vi "Error Query.vi"(8 "error in (no error)":errorcluster, 11 "VISA resource name":refnum<visa-resource-name>) -> (0 "error out":errorcluster, 1 "Error Message":string, 2 "Error Code":i32[](array[numeric]), 3 "VISA resource name out":refnum<visa-resource-name>)   [LabVIEW 2013]
doc: "This VI queries the instrument for any errors in the instrument's error queue. It will continue to read errors until all errors have been read from the instrument. Any errors will be returned in the Error Out cluster.\n\nNote:\nThis VI is called automatically by most driver VIs so it is not usually necessary to call this in an application."
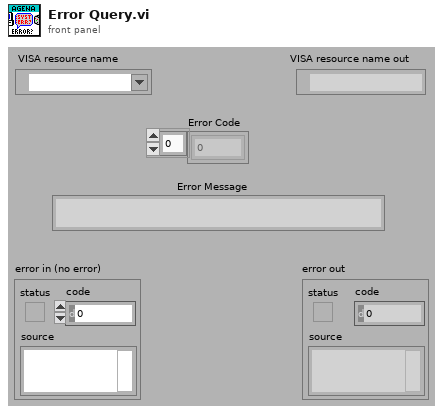
[diagram p1: front panel]
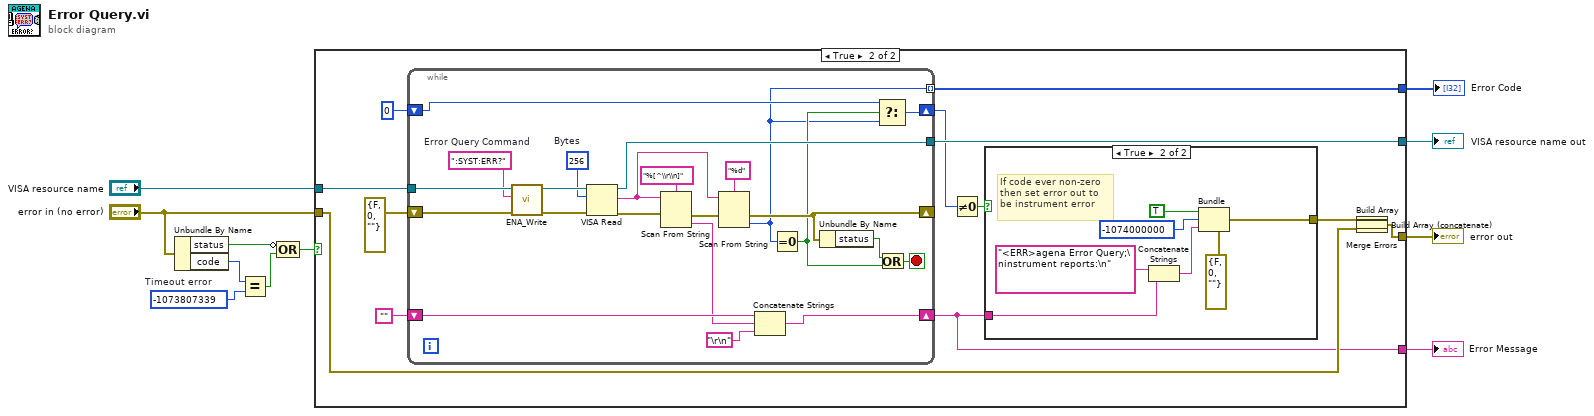
[diagram p0: block diagram]
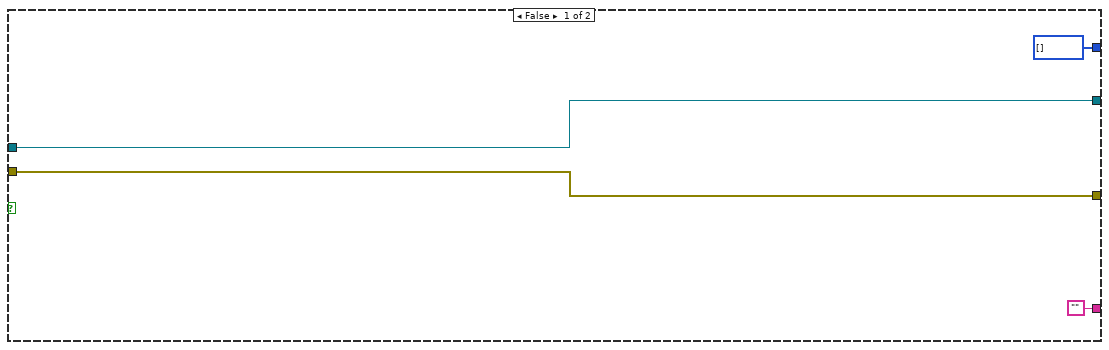
[diagram p2: hidden frame]
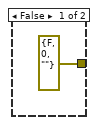
[diagram p3: hidden frame]
diagram:
  w6 = -1073807339  # Timeout error
  n1 = Unbundle By Name("error in (no error)") -> ("status"=w7:bool, "code"=w4:i32)
  n2 = Equal?(x=w4, y=w6) -> (x = y?=w5:bool)
  n3 = Compound Arithmetic op=OR(invert w7, w5) -> (w3:bool)
  n4 = case shown="True" w3 {
    tunnel: [w15 w29] -> w11
    tunnel: "VISA resource name" -> [w15 w28]
    tunnel: "error in (no error)" -> [w14 w22]
    tunnel: [w14 w26] -> w9
    tunnel: ["" w19] -> w2
    tunnel: [i32[] [] w18] -> w1
    frame False {
    }
    frame True {
      n5 = while {
        tunnel: [w60] -> w29
        tunnel: w28 -> [w59]
        shift-right: [w47] -> w19
        shift-left: "" -> [w50]
        shift-right: [w45] -> w20
        shift-left: 0 -> [w46]
        shift-right: [w43] -> _
        shift-left: errorcluster {"status"=FALSE, "code"=0, "source"=""} ("error in (no error)") -> [w44]
        tunnel: [w38] -> w18 mode=indexing
        stop <- w53 stop-if-true
        w57 = u32 256  # Bytes
        w55 = ":SYST:ERR?"  # Error Query Command
        n6 = call "ENA_Write.vi"("error in (no error)"=w44, "String ()"=w55, "VISA resource name"=w59) -> ("error out"=w56:errorcluster, "VISA resource name out"=w58:refnum<visa-resource-name>)  [unwired: 6 in, 1 out]
        n7 = VISA Read(VISA resource name=w58, byte count=w57, error in (no error)=w56) -> (VISA resource name out=w60:refnum<visa-resource-name>, read buffer=w51:string, error out=w42:errorcluster)  [unwired: 1 out]
        n8 = Scan From String(format string="%[^\\r\\n]", input string=w51, error in=w42) -> (error out=w41:errorcluster, output 1=w48:string)  [unwired: 2 in, 2 out]
        n9 = Scan From String(format string="%d", input string=w51, error in=w41) -> (error out=w43:errorcluster, output 1=w38:i32)  [unwired: 2 in, 2 out]
        n10 = Concatenate Strings(w50, w48, "\r\n") -> (w47:string)
        n11 = Equal To 0?(x=w38) -> (x = 0?=w39:bool)
        n12 = Unbundle By Name(w43) -> ("status"=w40:bool)
        n13 = Select(t=w46, s=w39, f=w38) -> (s? t:f=w45:i32)
        n14 = Or(x=w40, y=w39) -> (x .or. y?=w53:bool)
      }
      n15 = Not Equal To 0?(x=w20) -> (x != 0?=w24:bool)
      n16 = case shown="True" w24 {
        tunnel: w19 -> [_ w33]
        tunnel: [errorcluster {"status"=FALSE, "code"=0, "source"=""} ("error out") w32] -> w23
        frame False {
        }
        frame True {
          # "If code ever non-zero\nthen set error out to\nbe instrument error"
          n17 = Concatenate Strings("<ERR>agena Error Query;\ninstrument reports:\n" ("Source"), w33) -> (w34:string)
          n18 = Bundle(cluster=errorcluster {"status"=FALSE, "code"=0, "source"=""} ("error out"), "status"=TRUE ("Status"), "code"=-1074000000 ("Code"), "source"=w34) -> (w32:errorcluster)
        }
      }
      n19 = Build Array(w23, w22) -> (w17:errorcluster[])
      n20 = Build Array (concatenate)(w17) -> (w16:errorcluster[])
      n21 = Merge Errors(w16) -> (w26:errorcluster)
    }
  }
  "VISA resource name out" <- w11
  "error out" <- w9
  "Error Message" <- w2
  "Error Code" <- w1
